vi "Read Counts Till Next Common Shot HW.vi"(8 "error in (no error)":errorcluster, 11 "BME_DG_System in":refnum<class "BME_DG_System.lvclass">) -> (0 "error out":errorcluster, 1 "LC Multiple":i64, 2 "CountsRemains":i64, 3 "BME_DG_System out":refnum<class "BME_DG_System.lvclass">, 4 "Master Trigger Counter":i64)   [LabVIEW 2009, in "POLARIS BME DG.lvlib" / "BME_DG_System.lvclass"]
doc: "This VI reads trigger counter from master DG and calculates remaining trigger signals till common counter at all channels.\n\nOut parameter:\n - Counts Remains : remaining trigger counters till common shot\n - Master Trigger Counter : Last picked out trigger counte of master DG\n - LC Multiple : Least common multiple of all output modulo values\n\n\n---------------\n\nauthor: Alexander Kessler, Helmholtz-Institut-Jena \nmaintainer: Alexander Kessler: alexander.kessler@uni-jena.de\n\n\nLicense Agreement for this software:\n\nCopyright (C)\nHelmholtz-Institut-Jena\nFröbelsteg 3\n07743 Jena\nGermany\n\nContact: alexander.kessler@uni-jena.de\n\nThis program is free software; you can redistribute it and/or modify it under the terms of the GNU General Public License as published by the Free Software Foundation; either version 2 of the license, or (at your option) any later version.\n\nThis program is distributed in the hope that it will be useful, but WITHOUT ANY WARRANTY; without even the implied warranty of MERCHANTABILITY or FITNESS FOR A PARTICULAR PURPOSE. See the GNU General License for more details (http://www.gnu.org)."
uses:
  BME_DG_System.lvclass
  BME_DG_Base/BME_DG_Base.lvclass
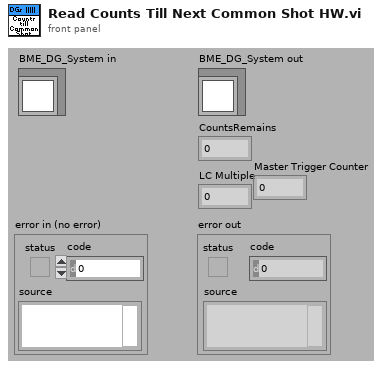
[diagram p1: front panel]
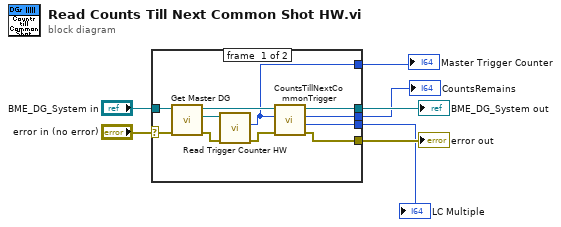
[diagram p0: block diagram]
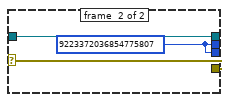
[diagram p2: hidden frame]
diagram:
  n1 = case shown="No Error" "error in (no error)" {
    selector: "error in (no error)" -> [w15 w21]
    tunnel: [w11 w21] -> w6
    tunnel: [w13 w20] -> w4
    tunnel: "BME_DG_System in" -> [w18 w20]
    tunnel: [w10 w19] -> w3
    tunnel: [w9 w19] -> w2
    tunnel: [w8 _] -> w1
    frame #0 {
      n2 = call "Get Master DG.vi"("error in (no error)"=w15, "BME_DG_System in"=w18) -> ("error out"=w17:errorcluster, "BME_DG_Base.lvclass"=w16:refnum<class "BME_DG_Base.lvclass">, "BME_DG_System out"=w14:refnum<class "BME_DG_System.lvclass">)  [unwired: 7 in]
      n3 = call "Read Trigger Counter HW.vi"("error in (no error)"=w17, "BME_DG_Base in"=w16) -> ("error out"=w12:errorcluster, "TriggerCounter"=w8:i64)  [unwired: 7 in, 1 out]
      n4 = call "CountsTillNextCommonTrigger.vi"("error in (no error)"=w12, "MasterTriggerCounter"=w8, "BME_DG_System in"=w14) -> ("error out"=w11:errorcluster, "LeastCommonMult"=w9:i64, "CountsRemains"=w10:i64, "BME_DG_System out"=w13:refnum<class "BME_DG_System.lvclass">)  [unwired: 5 in]
    }
    frame #1 {
      w19 = i64 9223372036854775807 ("CountsRemains")
    }
  }
  "error out" <- w6
  "BME_DG_System out" <- w4
  "CountsRemains" <- w3
  "LC Multiple" <- w2
  "Master Trigger Counter" <- w1
